vi "loadfile.vi"(8 "Error In":errorcluster) -> (0 "Error Out":errorcluster, 3 "Data":i64[](array[numeric]))   [LabVIEW 2023]
uses:
  <vilib>/Utility/file.llb/Read Delimited Spreadsheet (string).vi
  queue/Front Panel Message Queue.lvlib
panel:
  out "Num Channels":i32
  out "Data Cutted":string[](array[string])
  out "Cutted":string[](array[string])
  in  "transpose":bool
  in  "Selezione Colonna":i32
  in  "Righe da Eliminare":i32
  out "file":string[][](table)
  in  "load":bool
  in  "Stop":bool
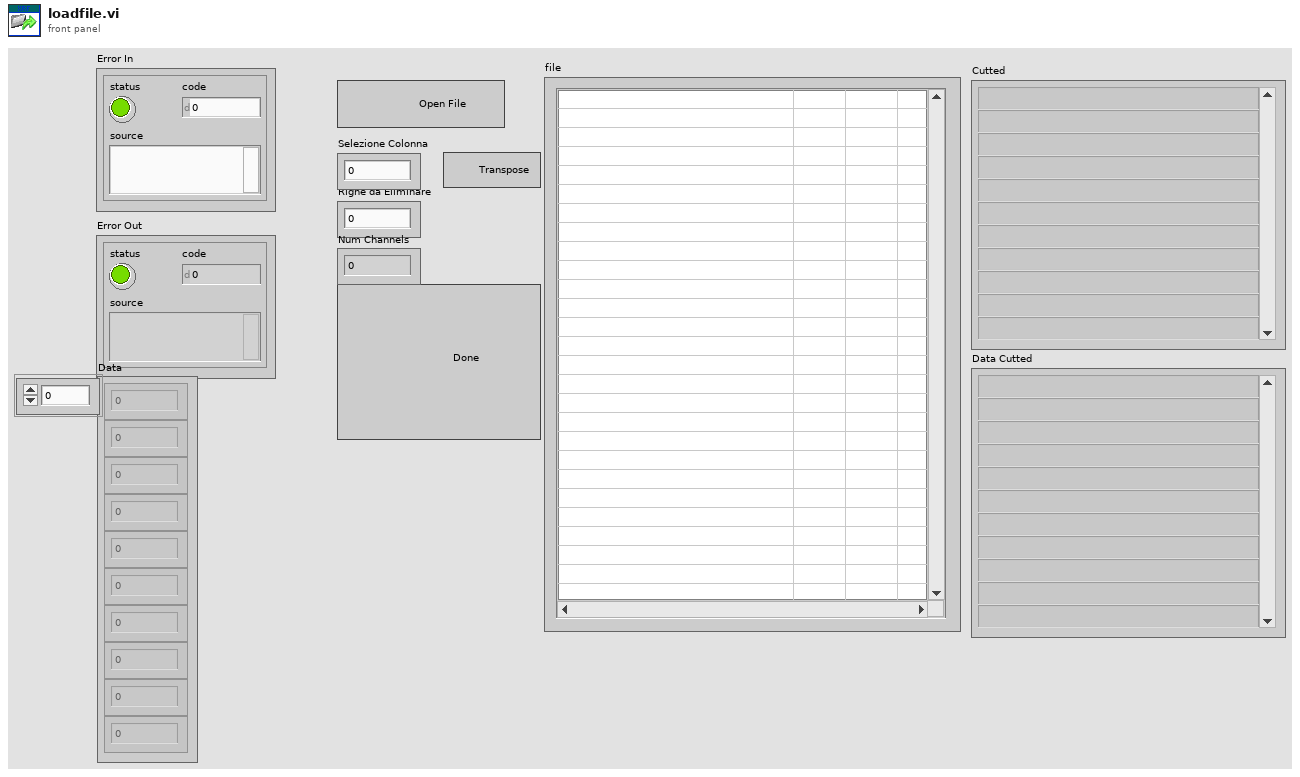
[diagram p1: front panel]
types:
  T1 = typedef "Front Panel Message Queue.lvlib/load Message Queues.ctl" = cluster{"Main":refnum<queue>}
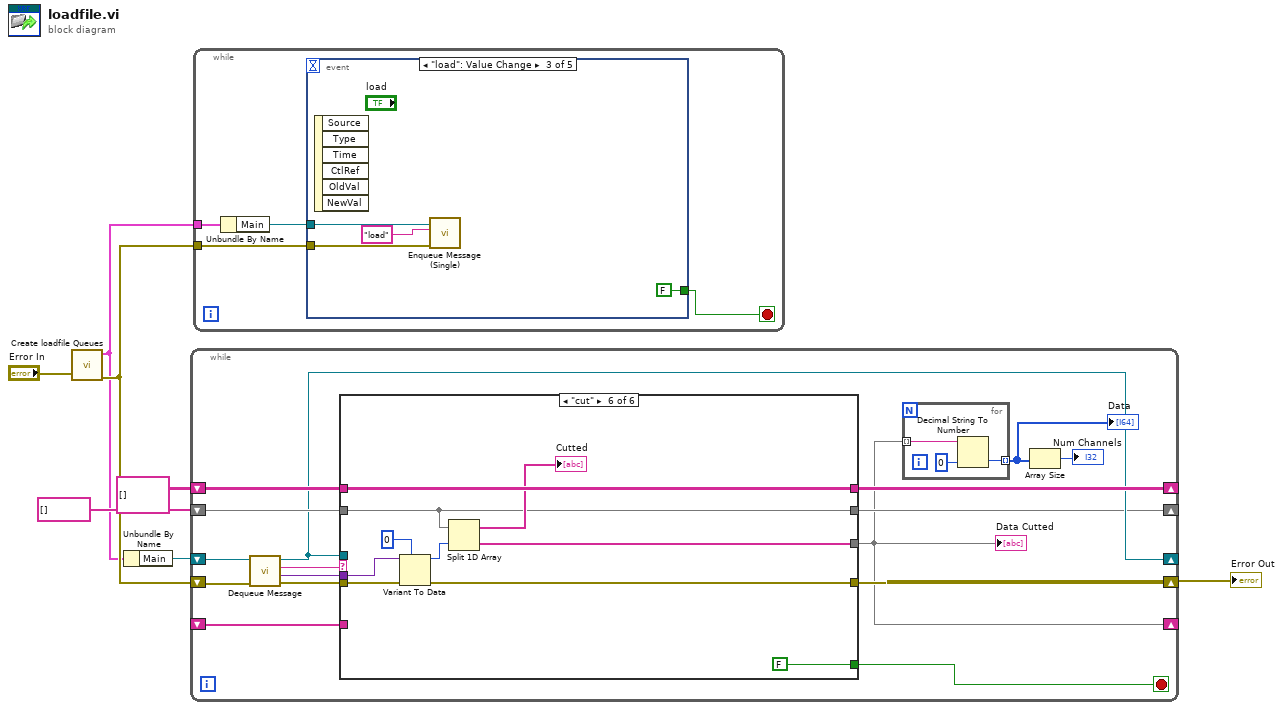
[diagram p0: block diagram]
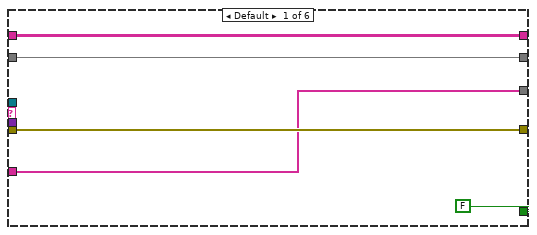
[diagram p2: hidden frame]
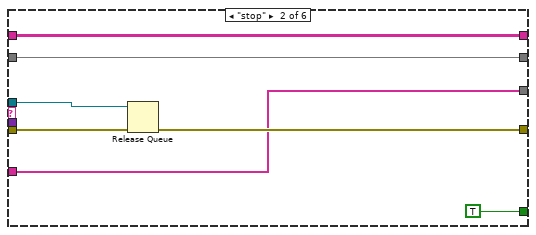
[diagram p3: hidden frame]
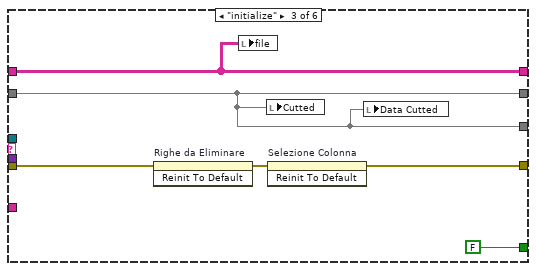
[diagram p4: hidden frame]
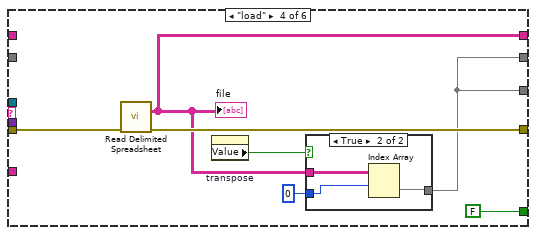
[diagram p5: hidden frame]
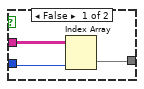
[diagram p6: hidden frame]
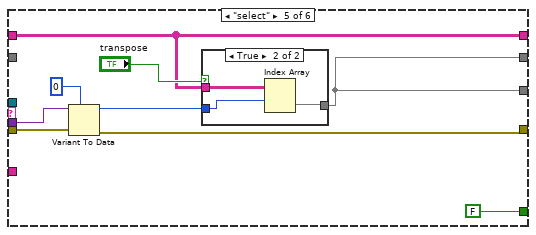
[diagram p7: hidden frame]
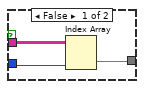
[diagram p8: hidden frame]
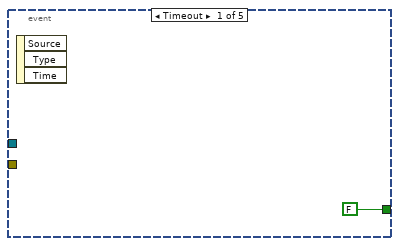
[diagram p9: hidden frame]
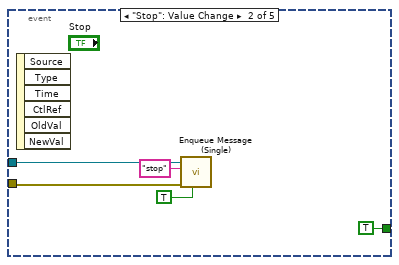
[diagram p10: hidden frame]
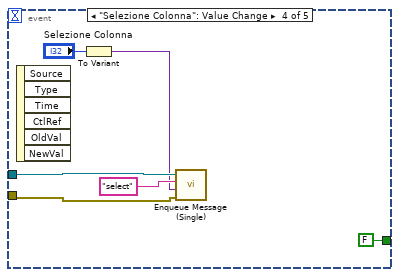
[diagram p11: hidden frame]
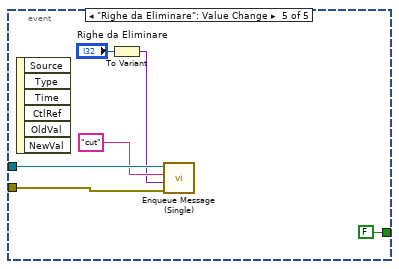
[diagram p12: hidden frame]
diagram:
  n1 = call "Create loadfile Queues.vi"("error in (no error)"="Error In") -> ("error out"=w6:errorcluster, "Message Queues"=w2:T1)  [unwired: 9 in]
  n2 = Unbundle By Name(w2) -> ("Main"=w1:refnum<queue>)
  n3 = while {
    shift-right: [w20] -> w5
    shift-left: w6 -> [w22]
    shift-right: [w18] -> _
    shift-left: string[][] [] ("all rows") -> [w17]
    shift-right: [w10] -> _
    shift-left: string[] [] ("all rows") -> [w15]
    shift-right: [w11] -> _
    shift-left: w1 -> [w12]
    shift-right: [w8] -> _
    shift-left: _ -> [w9]
    stop <- w19 stop-if-true
    n4 = call "Dequeue Message.vi"("error in (no error)"=w22, "Message Queue"=w12) -> ("error out"=w21:errorcluster, "Message Data"=w16:variant, "Message"=w23:string, "dup Message Queue"=w11:refnum<queue>)  [unwired: 5 in, 1 out]
    n5 = case shown="\"cut\"" w23 {
      tunnel: w21 -> [w31 w38 w41 w50 w65 w81]
      tunnel: [w31 w37 w40 w49 w61 w77] -> w20
      tunnel: [FALSE TRUE FALSE FALSE FALSE FALSE] -> w19
      tunnel: w11 -> [_ w35 _ _ _ _]
      tunnel: [w29 w34 w43 w47 w59 w76] -> w18
      tunnel: w17 -> [w29 w34 w43 _ w59 w76]
      tunnel: w16 -> [_ _ _ _ w64 w80]
      tunnel: [w27 w32 w39 w45 w58 w74] -> w8
      tunnel: w15 -> [w28 w33 w39 _ _ w73]
      tunnel: [w28 w33 w39 w45 w58 w73] -> w10
      tunnel: w9 -> [w27 w32 _ _ _ _]
      frame Default {
      }
      frame "stop" {
        n6 = Release Queue(queue=w35, error in (no error)=w38) -> (error out=w37:errorcluster)  [unwired: 1 in, 2 out]
      }
      frame "initialize" {
        n7 = invoke on="Righe da Eliminare" class="DigNum (strict)" method="Reinit To Default"(error in=w41) -> (error out=w42:errorcluster)  [unwired: 2 in, 2 out]
        n8 = local write "file"(w43) -> ()
        n9 = local write "Cutted"(w39) -> ()
        n10 = invoke on="Selezione Colonna" class="DigNum (strict)" method="Reinit To Default"(error in=w42) -> (error out=w40:errorcluster)  [unwired: 2 in, 2 out]
        n11 = local write "Data Cutted"(w39) -> ()
      }
      frame "load" {
        n12 = call-poly <vilib>:"Read Delimited Spreadsheet.vi"("error in (no error)"=w50) -> ("all rows"=w47:string[][], "error out"=w49:errorcluster)  [unwired: 9 in, 4 out]
        "file" <- w47
        n13 = property on="transpose" class="Bool (strict)"() -> ("Value"=w48:bool)  [unwired: 2 in, 2 out]
        n14 = case shown="True" w48 {
          tunnel: w47 -> [w54 w57]
          tunnel: 0 ("index (row)") -> [w53 w56]
          tunnel: [w52 w55] -> w45
          frame False {
            n15 = Index Array(array=w54, index (col)=w53) -> (element=w52:string[])  [unwired: 1 in]
          }
          frame True {
            n16 = Index Array(array=w57, index (row)=w56) -> (element=w55:string[])  [unwired: 1 in]
          }
        }
      }
      frame "select" {
        n17 = Variant To Data(error in=w65, type=0, Variant=w64) -> (data=w62:i32, error out=w61:errorcluster)
        n18 = case shown="True" "transpose" {
          tunnel: w59 -> [w69 w72]
          tunnel: w62 -> [w68 w71]
          tunnel: [w67 w70] -> w58
          frame False {
            n19 = Index Array(array=w69, index (col)=w68) -> (element=w67:string[])  [unwired: 1 in]
          }
          frame True {
            n20 = Index Array(array=w72, index (row)=w71) -> (element=w70:string[])  [unwired: 1 in]
          }
        }
      }
      frame "cut" {
        n21 = Variant To Data(error in=w81, type=0, Variant=w80) -> (data=w78:i32, error out=w77:errorcluster)
        n22 = Split 1D Array(array=w73, index=w78) -> (first subarray=→"Cutted":string[], second subarray=w74:string[])
      }
    }
    "Data Cutted" <- w8
    n23 = for {
      tunnel: w8 -> [w26] mode=indexing
      tunnel: [w25] -> w13 mode=indexing
      n24 = Decimal String To Number(string=w26, default (0L)=i64 0 ("default (0 I32)")) -> (number=w25:i64)  [unwired: 1 in, 1 out]
    }
    "Data" <- w13
    n25 = Array Size(array=w13) -> (size(s)=→"Num Channels":i32)
  }
  "Error Out" <- w5
  n26 = while {
    tunnel: w2 -> [w85]
    tunnel: w6 -> [w86]
    stop <- w83 stop-if-true
    n27 = Unbundle By Name(w85) -> ("Main"=w84:refnum<queue>)
    n28 = event shown="[2] \"load\": Value Change" {
      selector: _ -> [_ _ _ _ _]
      dyn-events: _ -> [_ _ _ _ _]
      timeout: _ -> [_ _ _ _ _]
      tunnel: w86 -> [_ w91 w94 w100 w107]
      tunnel: w84 -> [_ w90 w93 w99 w106]
      tunnel: [FALSE TRUE FALSE FALSE FALSE] -> w83
      event Timeout {
        n29 = event-data() -> ()  [unwired: 1 in, 3 out]
      }
      event "Stop": Value Change {
        n30 = event-data() -> ()  [unwired: 1 in, 6 out]
        n31 = call "Enqueue Message (Single).vi"("Priority Message? (F)"=TRUE, "error in (no error)"=w91, "Message"="stop", "Message Queue"=w90) -> ()  [unwired: 6 in, 2 out]
      }
      event "load": Value Change {
        n32 = event-data() -> ()  [unwired: 1 in, 6 out]
        n33 = call "Enqueue Message (Single).vi"("error in (no error)"=w94, "Message"="load", "Message Queue"=w93) -> ()  [unwired: 7 in, 2 out]
      }
      event "Selezione Colonna": Value Change {
        n34 = event-data() -> ()  [unwired: 1 in, 6 out]
        n35 = To Variant(anything="Selezione Colonna") -> (Variant=w97:variant)
        n36 = call "Enqueue Message (Single).vi"("error in (no error)"=w100, "Message Data"=w97, "Message"="select", "Message Queue"=w99) -> ()  [unwired: 6 in, 2 out]
      }
      event "Righe da Eliminare": Value Change {
        n37 = event-data() -> ()  [unwired: 1 in, 6 out]
        n38 = To Variant(anything="Righe da Eliminare") -> (Variant=w103:variant)
        n39 = call "Enqueue Message (Single).vi"("error in (no error)"=w107, "Message Data"=w103, "Message"="cut", "Message Queue"=w106) -> ()  [unwired: 6 in, 2 out]
      }
    }
  }
